vi "SP Convert 1.3 - 1.4 to 1.5.vi"(1 "S Parameter 1.3 - 1.4 Test Parameters":T2 {"Stimulus"."Sweep Time, s" format="%.3g"; "Measurements"."Channel (CH 1)" items=["CH 1", "CH 2", "CH 3", "CH 4"]}) -> (0 "S Parameter 1.5 Test Parameters":T1={"Tag"="", "Calibration"=enum."Not Calibrated", "Stimulus"={"Use Instrument Settings"=FALSE, "Sweep Type"=enum."Linear", "Sweep"=[], "Blank Frequencies"=FALSE, "Power, dBm"=0.0, "IFBW, Hz"=0.0, "Sweep Time, s"=0.0}, "Measurements"=[], "Reports"={"Reports to Generate"=[], "Print Reports"=TRUE}, "Quick Mode"=FALSE} {"Stimulus"."Sweep Time, s" format="%.3g"; "Measurements"."Channel (CH 1)" items=["CH 1", "CH 2", "CH 3", "CH 4"]})   [LabVIEW 2011]
uses:
  TypeDefs/SP Test Parameters v1.3-1.4.ctl
  TypeDefs/SP Test Parameters v1.5.ctl
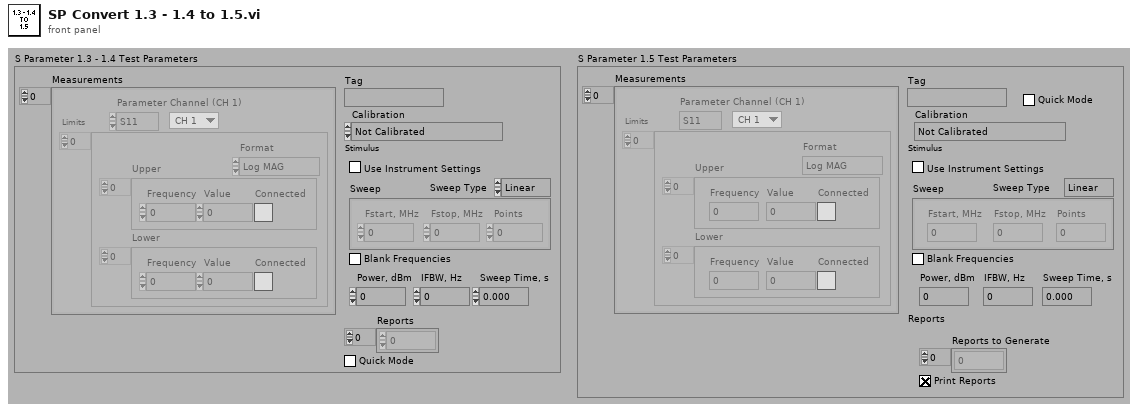
[diagram p1: front panel]
types:
  T1 = typedef "SP Test Parameters v1.5.ctl" = cluster{"Tag":string, "Calibration":enum32{"Not Calibrated", "Response", "Response and Isolation", "Full 1-Port (Port 1)", "Full 1-Port (Port 2)", "Full 2-Port", "One Path 2-Port", "TRL/LRM  2-Port"}, "Stimulus":cluster{"Use Instrument Settings":bool, "Sweep Type":enum32{"Linear", "Log", "List", "Power", "CW"}, "Sweep":cluster{"Fstart, MHz":dbl, "Fstop, MHz":dbl, "Points":i32}[], "Blank Frequencies":bool, "Power, dBm":dbl, "IFBW, Hz":dbl, "Sweep Time, s":dbl}, "Measurements":cluster{"Parameter":enum32{"S11", "S21", "S12", "S22"}, "Limits":cluster{"Format":enum16{"Log MAG", "Lin MAG", "VSWR", "Phase", "Delay", "Insertion Loss", "Isolation", "Return Loss"}, "Upper":cluster{"Frequency":dbl, "Value":dbl, "Connected":bool}[], "Lower":cluster{"Frequency":dbl, "Value":dbl, "Connected":bool}[]}[], "Channel (CH 1)":u16}[], "Reports":cluster{"Reports to Generate":i32[], "Print Reports":bool}, "Quick Mode":bool}
  T2 = typedef "SP Test Parameters v1.3-1.4.ctl" = cluster{"Tag":string, "Calibration":enum32{"Not Calibrated", "Response", "Response and Isolation", "Full 1-Port (Port 1)", "Full 1-Port (Port 2)", "Full 2-Port", "One Path 2-Port", "TRL/LRM  2-Port"}, "Stimulus":cluster{"Use Instrument Settings":bool, "Sweep Type":enum32{"Linear", "Log", "List", "Power", "CW"}, "Sweep":cluster{"Fstart, MHz":dbl, "Fstop, MHz":dbl, "Points":i32}[], "Blank Frequencies":bool, "Power, dBm":dbl, "IFBW, Hz":dbl, "Sweep Time, s":dbl}, "Measurements":cluster{"Parameter":enum32{"S11", "S21", "S12", "S22"}, "Limits":cluster{"Format":enum16{"Log MAG", "Lin MAG", "VSWR", "Phase", "Delay", "Insertion Loss", "Isolation", "Return Loss"}, "Upper":cluster{"Frequency":dbl, "Value":dbl, "Connected":bool}[], "Lower":cluster{"Frequency":dbl, "Value":dbl, "Connected":bool}[]}[], "Channel (CH 1)":u16}[], "Reports":i32[], "Quick Mode":bool}
  T3 = enum32{"Not Calibrated", "Response", "Response and Isolation", "Full 1-Port (Port 1)", "Full 1-Port (Port 2)", "Full 2-Port", "One Path 2-Port", "TRL/LRM  2-Port"}
  T4 = cluster{"Use Instrument Settings":bool, "Sweep Type":enum32{"Linear", "Log", "List", "Power", "CW"}, "Sweep":cluster{"Fstart, MHz":dbl, "Fstop, MHz":dbl, "Points":i32}[], "Blank Frequencies":bool, "Power, dBm":dbl, "IFBW, Hz":dbl, "Sweep Time, s":dbl}
  T5 = cluster{"Parameter":enum32{"S11", "S21", "S12", "S22"}, "Limits":cluster{"Format":enum16{"Log MAG", "Lin MAG", "VSWR", "Phase", "Delay", "Insertion Loss", "Isolation", "Return Loss"}, "Upper":cluster{"Frequency":dbl, "Value":dbl, "Connected":bool}[], "Lower":cluster{"Frequency":dbl, "Value":dbl, "Connected":bool}[]}[], "Channel (CH 1)":u16}[]
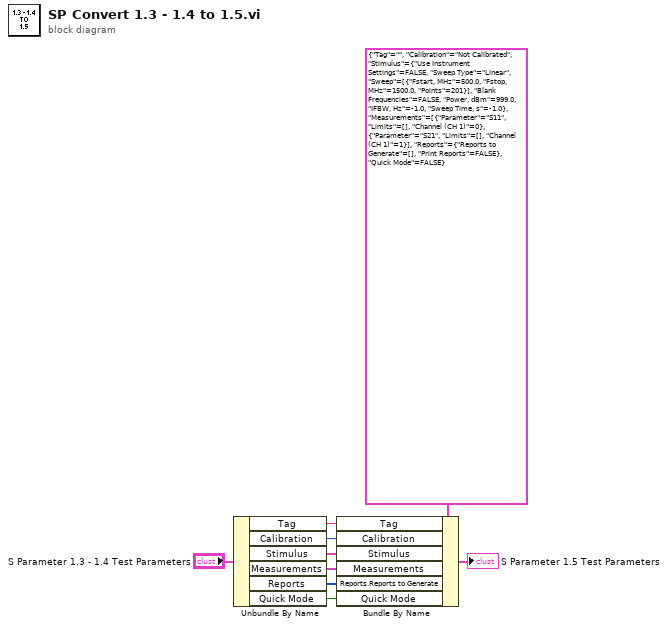
[diagram p0: block diagram]
diagram:
  n1 = Unbundle By Name("S Parameter 1.3 - 1.4 Test Parameters") -> ("Tag"=w6:string, "Calibration"=w5:T3, "Stimulus"=w4:T4, "Measurements"=w3:T5, "Reports"=w1:i32[], "Quick Mode"=w2:bool)
  n2 = Bundle By Name(cluster=T1 {"Tag"="", "Calibration"=enum."Not Calibrated", "Stimulus"={"Use Instrument Settings"=FALSE, "Sweep Type"=enum."Linear", "Sweep"=[{"Fstart, MHz"=500.0, "Fstop, MHz"=1500.0, "Points"=201}], "Blank Frequencies"=FALSE, "Power, dBm"=999.0, "IFBW, Hz"=-1.0, "Sweep Time, s"=-1.0}, "Measurements"=[{"Parameter"=enum."S11", "Limits"=[], "Channel (CH 1)"=0}, {"Parameter"=enum."S21", "Limits"=[], "Channel (CH 1)"=1}], "Reports"={"Reports to Generate"=[], "Print Reports"=FALSE}, "Quick Mode"=FALSE} ("S Parameter Test Parameters"), "Tag"=w6, "Calibration"=w5, "Stimulus"=w4, "Measurements"=w3, "Reports.Reports to Generate"=w1, "Quick Mode"=w2) -> (→"S Parameter 1.5 Test Parameters":T1)
